vi "IsArmed.vi"(8 "error in (no error)":errorcluster, 11 "Red Pitaya Digitizer in":refnum<class "Red Pitaya Digitizer.lvclass">) -> (0 "error out":errorcluster, 1 "Finished":bool, 2 "Armed":bool, 3 "Red Pitaya Digitizer out":refnum<class "Red Pitaya Digitizer.lvclass">, 4 "Availiable Samples":u32)   [LabVIEW 2015, in "Red Pitaya Digitizer.lvclass"]
uses:
  Red Pitaya Digitizer.lvclass
  Red Pitaya Digitizer.lvclass/Red Pitaya Digitizer.ctl
  Read RP Instrument.vi
  Write RP Instrument.vi
  RP Core/RP Instrument/RP Instrument.lvclass
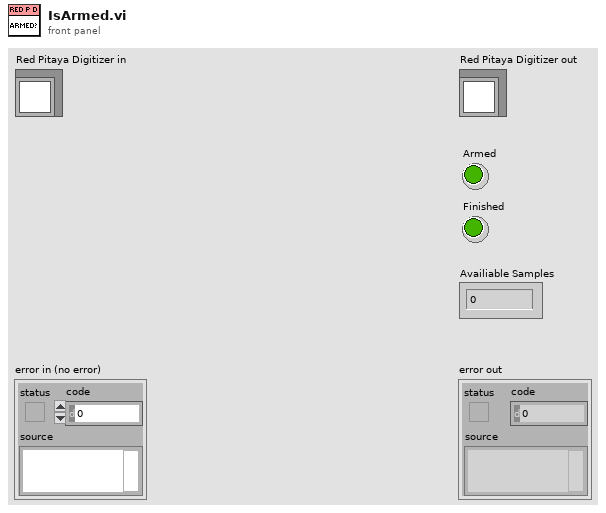
[diagram p1: front panel]
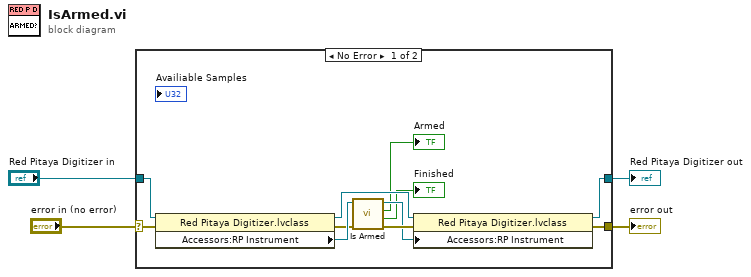
[diagram p0: block diagram]
diagram:
  n1 = case shown="No Error" "error in (no error)" {
    selector: "error in (no error)" -> [w12 w17]
    tunnel: "Red Pitaya Digitizer in" -> [w15 w16]
    tunnel: [w8 w16] -> w2
    tunnel: [w7 w17] -> w1
    frame No Error {
      n2 = property class="Red Pitaya Digitizer.lvclass"(reference=w15, error in=w12) -> (reference out=w11:refnum<class "Red Pitaya Digitizer.lvclass">, error out=w13:errorcluster, "Accessors:RP Instrument"=w14:refnum<class "RP Instrument.lvclass">)
      n3 = call-dynamic "Is Armed.vi"("error in (no error)"=w13, "RP Instrument in"=w14) -> ("error out"=w10:errorcluster, "Finished"=→"Finished":bool, "Armed"=→"Armed":bool, "RP Instrument out"=w9:refnum<class "RP Instrument.lvclass">)  [unwired: 6 in]
      n4 = property class="Red Pitaya Digitizer.lvclass"(reference=w11, error in=w10, "Accessors:RP Instrument"=w9) -> (reference out=w8:refnum<class "Red Pitaya Digitizer.lvclass">, error out=w7:errorcluster)
    }
    frame Error {
    }
  }
  "error out" <- w1
  "Red Pitaya Digitizer out" <- w2
